vi "Polar Plot - Font Type (Write Property).vi"(5 "Value":T1(ring), 6 "Container State":T2, 7 "Display State In":T3={"Plot Attributes"={"maximum"=2.0, "minimum"=0.0, "clip to min"=FALSE, "log"=FALSE, "grid color"=3381657, "plot color"=16711680, "fmt and prec"={"format"=enum."Decimal", "precision"=2}, "visible section"=4}, "Desired Font"=enum."Application Font", "User-Specified Font"={"Font Name:"="Arial", "Size"=9, "Strikeout?"=FALSE, "Italic?"=FALSE, "Underline?"=FALSE, "Outline?"=FALSE, "Shadow?"=FALSE, "Bold?"=FALSE}} {"Plot Attributes"."minimum" format="%0.2f"; "Plot Attributes"."maximum" format="%0.2f"}) -> (0 "error out":errorcluster, 3 "Display State Out":T3={"Plot Attributes"={"maximum"=2.0, "minimum"=0.0, "clip to min"=FALSE, "log"=FALSE, "grid color"=3381657, "plot color"=16711680, "fmt and prec"={"format"=enum."Decimal", "precision"=2}, "visible section"=4}, "Desired Font"=enum."Application Font", "User-Specified Font"={"Font Name:"="Arial", "Size"=9, "Strikeout?"=FALSE, "Italic?"=FALSE, "Underline?"=FALSE, "Outline?"=FALSE, "Shadow?"=FALSE, "Bold?"=FALSE}} {"Plot Attributes"."minimum" format="%0.2f"; "Plot Attributes"."maximum" format="%0.2f"})   [LabVIEW 2009, in "Polar Plot.xctl"]
doc: "Demonstration of an XControl.\n\nAAL 9/09"
uses:
  Polar Plot.xctl
  Abilities/Polar Plot - State.ctl
  <vilib>/_xctls/Container State.ctl
  <vilib>/_xctls/XControlSupport.lvlib
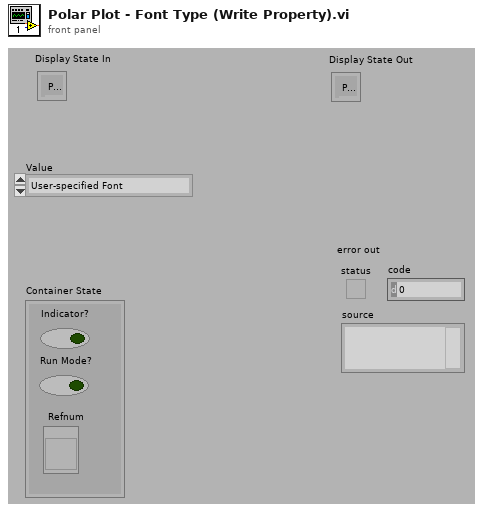
[diagram p1: front panel]
types:
  T1 = enum16{"User-specified Font", "Application Font", "System Font", "Dialog Font"}
  T2 = typedef "XControlSupport.lvlib/Container State.ctl" = cluster{"Indicator?":bool, "Run Mode?":bool, " Refnum":refnum<vi>}
  T3 = typedef "Polar Plot.xctl/Polar Plot - State.ctl" = cluster{"Plot Attributes":cluster{"maximum":dbl, "minimum":dbl, "clip to min":bool, "log":bool, "grid color":u32, "plot color":u32, "fmt and prec":cluster{"format":enum8{"Decimal", "Scientific", "Engineering", "Binary", "Octal", "Hex"}, "precision":u8}, "visible section":u16}, "Desired Font":enum16{"User-specified Font", "Application Font", "System Font", "Dialog Font"}, "User-Specified Font":cluster{"Font Name:":string, "Size":i16, "Strikeout?":bool, "Italic?":bool, "Underline?":bool, "Outline?":bool, "Shadow?":bool, "Bold?":bool}}
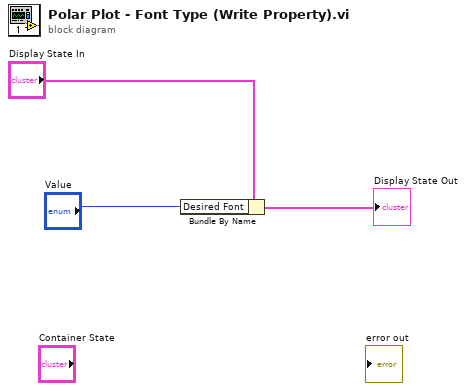
[diagram p0: block diagram]
diagram:
  n1 = Bundle By Name(cluster="Display State In", "Desired Font"="Value") -> (→"Display State Out":T3)
